vi "String to Array Test.vi"(8 "Error In":errorcluster) -> (0 "Error Out":errorcluster)   [LabVIEW 2019, in "Test.lvlib"]
doc: "The VI is a test file that tests the functionality of conversion of string to array with and without spaces."
uses:
  Test.lvlib
  <vilib>/addons/_JKI Toolkits/Caraya/classes/Assert/Assert.lvclass
  <vilib>/addons/_JKI Toolkits/Caraya/classes/Assert/Assert Equal Value_Variant.vi
  <vilib>/addons/_JKI Toolkits/Caraya/classes/Test/Test.lvclass
  File Path Operations/File and Path Operations.lvlib
panel:
  # "STRING TO ARRAY TEST"
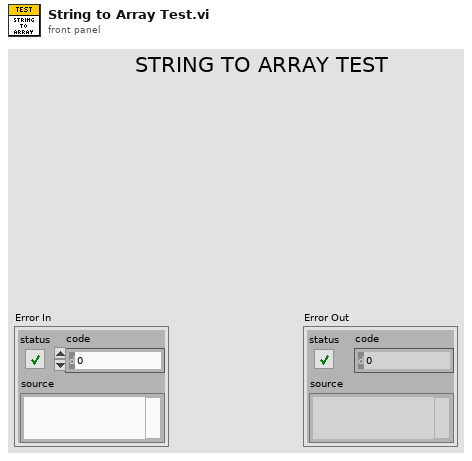
[diagram p1: front panel]
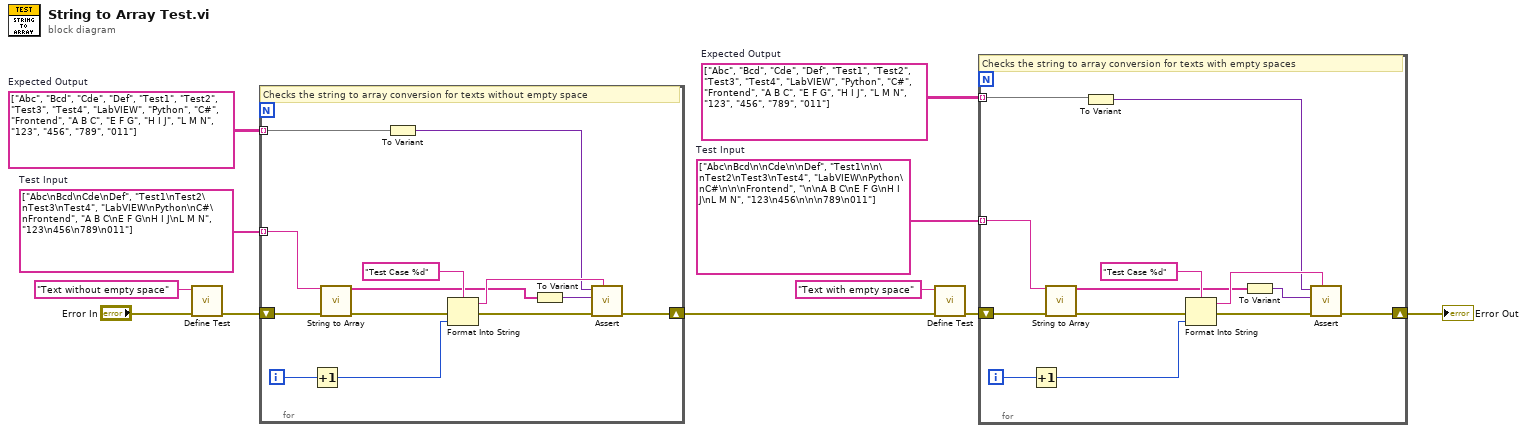
[diagram p0: block diagram]
diagram:
  w1 = string[][] [["Abc", "Bcd", "Cde", "Def"], ["Test1", "Test2", "Test3", "Test4"], ["LabVIEW", "Python", "C#", "Frontend"], ["A B C", "E F G", "H I J", "L M N"], ["123", "456", "789", "011"]]  # Expected Output
  w2 = string[] ["Abc\nBcd\n\nCde\n\nDef", "Test1\n\n\nTest2\nTest3\nTest4", "LabVIEW\nPython\nC#\n\n\nFrontend", "\n\nA B C\nE F G\nH I J\nL M N", "123\n456\n\n\n789\n011"]  # Test Input
  w7 = string[][] [["Abc", "Bcd", "Cde", "Def"], ["Test1", "Test2", "Test3", "Test4"], ["LabVIEW", "Python", "C#", "Frontend"], ["A B C", "E F G", "H I J", "L M N"], ["123", "456", "789", "011"]]  # Expected Output
  w8 = string[] ["Abc\nBcd\nCde\nDef", "Test1\nTest2\nTest3\nTest4", "LabVIEW\nPython\nC#\nFrontend", "A B C\nE F G\nH I J\nL M N", "123\n456\n789\n011"]  # Test Input
  n1 = call <vilib>:"Define Test.vi"("error in (no error)"="Error In", "Label (VI Title)"="Text without empty space") -> ("error out"=w9:errorcluster)  [unwired: 8 in, 1 out]
  n2 = for {
    shift-right: [w18] -> w4
    shift-left: w9 -> [w17]
    tunnel: w8 -> [w14] mode=indexing
    tunnel: w7 -> [w19] mode=indexing
    i -> [w23]
    # "Checks the string to array conversion for texts without empty space"
    n3 = Increment(x=w23) -> (x+1=w20:i32)
    n4 = call "String to Array.vi"("Input String"=w14, "Error In"=w17) -> ("Array of Strings"=w15:string[], "Error Out"=w16:errorcluster)  [unwired: 12 in]
    n5 = To Variant(anything=w19) -> (Variant=w13:variant)
    n6 = Format Into String(format string="Test Case %d", error in=w16, w20) -> (resulting string=w21:string, error out=w24:errorcluster)  [unwired: 1 in]
    n7 = To Variant(anything=w15) -> (Variant=w12:variant)
    n8 = call-poly <vilib>:"Assert.vi"("Label"=w21, "error in (no error)"=w24, "Y"=w12, "X"=w13) -> ("error out"=w18:errorcluster)  [unwired: 6 in, 1 out]
  }
  n9 = call <vilib>:"Define Test.vi"("error in (no error)"=w4, "Label (VI Title)"="Text with empty space") -> ("error out"=w5:errorcluster)  [unwired: 8 in, 1 out]
  n10 = for {
    shift-right: [w32] -> w3
    shift-left: w5 -> [w31]
    tunnel: w2 -> [w28] mode=indexing
    tunnel: w1 -> [w27] mode=indexing
    i -> [w36]
    # "Checks the string to array conversion for texts with empty spaces"
    n11 = Increment(x=w36) -> (x+1=w33:i32)
    n12 = call "String to Array.vi"("Input String"=w28, "Error In"=w31) -> ("Array of Strings"=w29:string[], "Error Out"=w30:errorcluster)  [unwired: 12 in]
    n13 = To Variant(anything=w27) -> (Variant=w25:variant)
    n14 = Format Into String(format string="Test Case %d", error in=w30, w33) -> (resulting string=w34:string, error out=w37:errorcluster)  [unwired: 1 in]
    n15 = To Variant(anything=w29) -> (Variant=w26:variant)
    n16 = call-poly <vilib>:"Assert.vi"("Label"=w34, "error in (no error)"=w37, "Y"=w26, "X"=w25) -> ("error out"=w32:errorcluster)  [unwired: 6 in, 1 out]
  }
  "Error Out" <- w3
